vi "Mapping Countdown v10.6.3.vi"(6 "Execution Times (s)":dbl[](array[numeric]), 9 "Mapping Spectra Settings":T1={"Integration Time"=10.0, "Repetitions"=10, "Mapping Spectra"=TRUE} {"Repetitions" min=1 max=100 step=1; "Integration Time" min=0.5 max=6000.0 step=1.0 format="%.1f"}, 10 "Ready Steps":i32, 11 "Mapping Drive Parameters":T2={"X Start Position"=10.0, "X Stop Position"=10.0, "Y Start Position"=10.0, "Y Stop Position"=10.0, "Step Size"=10.0} {"Step Size" min=0.1 max=30.0 step=0.1 format="%.1f"; "Y Stop Position" min=0.0 max=30.0 step=0.1 format="%.1f"; "Y Start Position" min=0.0 max=30.0 step=0.1 format="%.1f"; "X Stop Position" min=0.0 max=30.0 step=0.1 format="%.1f"; "X Start Position" min=0.0 max=30.0 step=0.1 format="%.1f"}) -> (2 "Progress":i16, 3 "Time String":string)   [LabVIEW 2010]
uses:
  TypeDefs/Mapping Drive Params.ctl
  TypeDefs/Mapping Spectra Params.ctl
  <vilib>/Analysis/NI_AALBase.lvlib
panel:
  out "Step Time (s)":dbl
  out "Left Time (s)":dbl
  out "Left Steps":dbl
  out "Total Steps":dbl
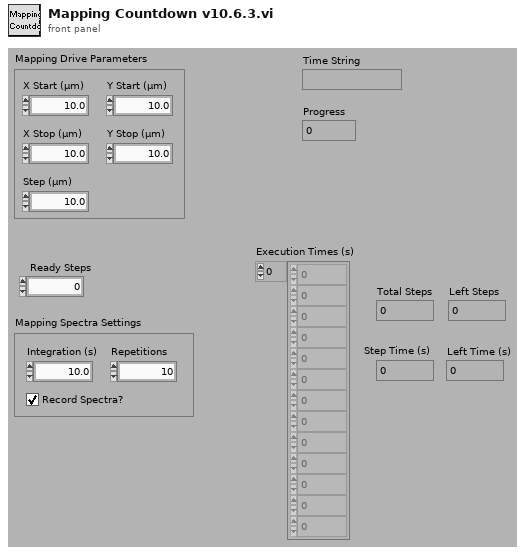
[diagram p1: front panel]
types:
  T1 = typedef "Mapping Spectra Params.ctl" = cluster{"Integration Time":dbl, "Repetitions":u16, "Mapping Spectra":bool}
  T2 = typedef "Mapping Drive Params.ctl" = cluster{"X Start Position":dbl, "X Stop Position":dbl, "Y Start Position":dbl, "Y Stop Position":dbl, "Step Size":dbl}
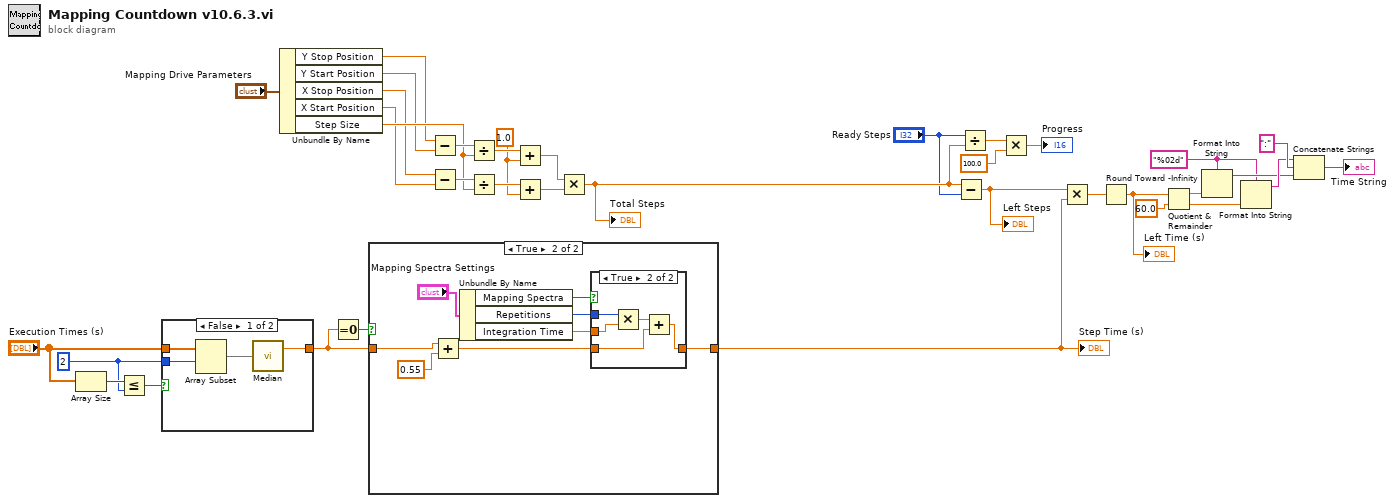
[diagram p0: block diagram]
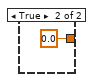
[diagram p2: hidden frame]
diagram:
  w4 = 2 ("index")
  w19 = 1.0 ("y")
  w31 = "%02d" ("Format-String")
  n1 = Array Size(array="Execution Times (s)") -> (size(s)=w7:i32)
  n2 = Less Or Equal?(x=w7, y=w4) -> (x <= y?=w6:bool)
  n3 = case shown="False" w6 {
    tunnel: "Execution Times (s)" -> [w39 _]
    tunnel: w4 -> [w38 _]
    tunnel: [w37 0.0 ("mean")] -> w3
    frame False {
      n4 = Array Subset(array=w39, index=w38) -> (w40:dbl[])  [unwired: 1 in]
      n5 = call <vilib>:"Median.vi"("X"=w40) -> ("median"=w37:dbl)  [unwired: 1 out]
    }
    frame True {
    }
  }
  n6 = Unbundle By Name("Mapping Drive Parameters") -> ("Y Stop Position"=w11:dbl, "Y Start Position"=w12:dbl, "X Stop Position"=w13:dbl, "X Start Position"=w14:dbl, "Step Size"=w15:dbl)
  n7 = Equal To 0?(x=w3) -> (x = 0?=w8:bool)
  n8 = case shown="True" w8 {
    tunnel: [w42 w45] -> w2
    tunnel: w3 -> [w42 w43]
    frame False {
    }
    frame True {
      n9 = Add(x=w43, y=0.55) -> (x+y=w44:dbl)
      n10 = Unbundle By Name("Mapping Spectra Settings") -> ("Mapping Spectra"=w48:bool, "Repetitions"=w47:u16, "Integration Time"=w46:dbl)
      n11 = case shown="True" w48 {
        tunnel: w47 -> [_ w56]
        tunnel: w46 -> [_ w55]
        tunnel: w44 -> [w51 w53]
        tunnel: [w51 w52] -> w45
        frame False {
        }
        frame True {
          n12 = Multiply(x=w56, y=w55) -> (x*y=w54:dbl)
          n13 = Add(x=w54, y=w53) -> (x+y=w52:dbl)
        }
      }
    }
  }
  "Step Time (s)" <- w2
  n14 = Subtract(x=w11, y=w12) -> (x-y=w23:dbl)
  n15 = Subtract(x=w13, y=w14) -> (x-y=w22:dbl)
  n16 = Divide(x=w23, y=w15) -> (x/y=w20:dbl)
  n17 = Divide(x=w22, y=w15) -> (x/y=w21:dbl)
  n18 = Add(x=w20, y=w19) -> (x+y=w10:dbl)
  n19 = Add(x=w21, y=w19) -> (x+y=w9:dbl)
  n20 = Multiply(x=w10, y=w9) -> (x*y=w18:dbl)
  "Total Steps" <- w18
  n21 = Subtract(x=w18, y="Ready Steps") -> (x-y=w17:dbl)
  "Left Steps" <- w17
  n22 = Divide(x="Ready Steps", y=w18) -> (x/y=w16:dbl)
  n23 = Multiply(x=w16, y=100.0) -> (x*y=→"Progress":dbl)
  n24 = Multiply(x=w17, y=w2) -> (x*y=w25:dbl)
  n25 = Round Toward -Infinity(1:w25) -> (0:w28:dbl)
  "Left Time (s)" <- w28
  n26 = Quotient & Remainder(x=w28, y=60.0) -> (x-y*floor(x/y)=w30:dbl, floor(x/y)=w29:dbl)
  n27 = Format Into String(format string=w31, w30) -> (resulting string=w32:string)  [unwired: 2 in, 1 out]
  n28 = Format Into String(format string=w31, w29) -> (resulting string=w33:string)  [unwired: 2 in, 1 out]
  n29 = Concatenate Strings(w33, ":" ("String"), w32) -> (→"Time String":string)
